vi "yolov10.vi"   [LabVIEW 2021]
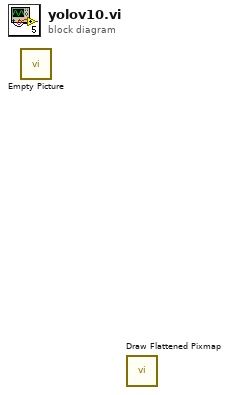
[diagram p0: block diagram]
diagram:
  n1 = call "Empty Picture"() -> ()  [unwired: 1 out]
  n2 = call <vilib>:"Draw Flattened Pixmap.vi"() -> ()  [unwired: 9 in, 1 out]
